vi "2013_04_30 Each Motor.vi"(6 "Temp On":dbl=1.0, 8 "Motor #":i32=1, 9 "data":waveform(dbl)[](array[waveform]), 10 "File Path":path=path "Durability/.lvm", 11 "Motor Typedef":T1 {"Elec Power In (W)" format="%.3g"; "Efficiency" format="%#_3g%%"; "Mech Pwr Out (W)" format="%.3g"; "Torque (mNm)" format="%.3g"; "Elapsed Time (h)" format="%.1f"; "Supply (V)" format="%.2f"; "RPM" scale=0.0..40000.0 scale format="%#_4p"}) -> (0 "Final Out":dynamicdata(graph), 1 "Counter":dbl, 3 "Motor Typedef Out":T1={"Enabled"=FALSE, "Fail"=FALSE, "RPM"=0.0, "Motor"=enum."Maxon EC6 6V", "ESC"=enum."Phoenix", "Supply (V)"=0.0, "Test ID and Serial #"="", "Comments"="", "Elapsed Time (h)"=0.0, "Counter"=0.0, "Torque (mNm)"=0.0, "Mech Pwr Out (W)"=0.0, "Efficiency"=0.0, "Elec Power In (W)"=0.0} {"Elec Power In (W)" format="%.3g"; "Efficiency" format="%#_3g%%"; "Mech Pwr Out (W)" format="%.3g"; "Torque (mNm)" format="%.3g"; "Elapsed Time (h)" format="%.1f"; "Supply (V)" format="%.2f"; "RPM" scale=0.0..40000.0 scale format="%#_4p"})   [LabVIEW 2013]
uses:
  MotorTypeDef.ctl
  <vilib>/express/express shared/transition.llb/Dynamic To Waveform Array.vi
  <vilib>/express/express signal manip/GetorSetDDTAttributes/Set DDT Attributes/SetT0.vi
  <vilib>/express/express shared/transition.llb/Waveform Array To Dynamic.vi
  <vilib>/express/express signal manip/GetorSetDDTAttributes/Set DDT Attributes/Set DDT Properties.xnode
panel:
  in  "error in (no error)":errorcluster
  out "error out":errorcluster
  out "Saving Data":bool
  # "Enable"
  # "Fail"
  # "Enable"
  # "Fail"
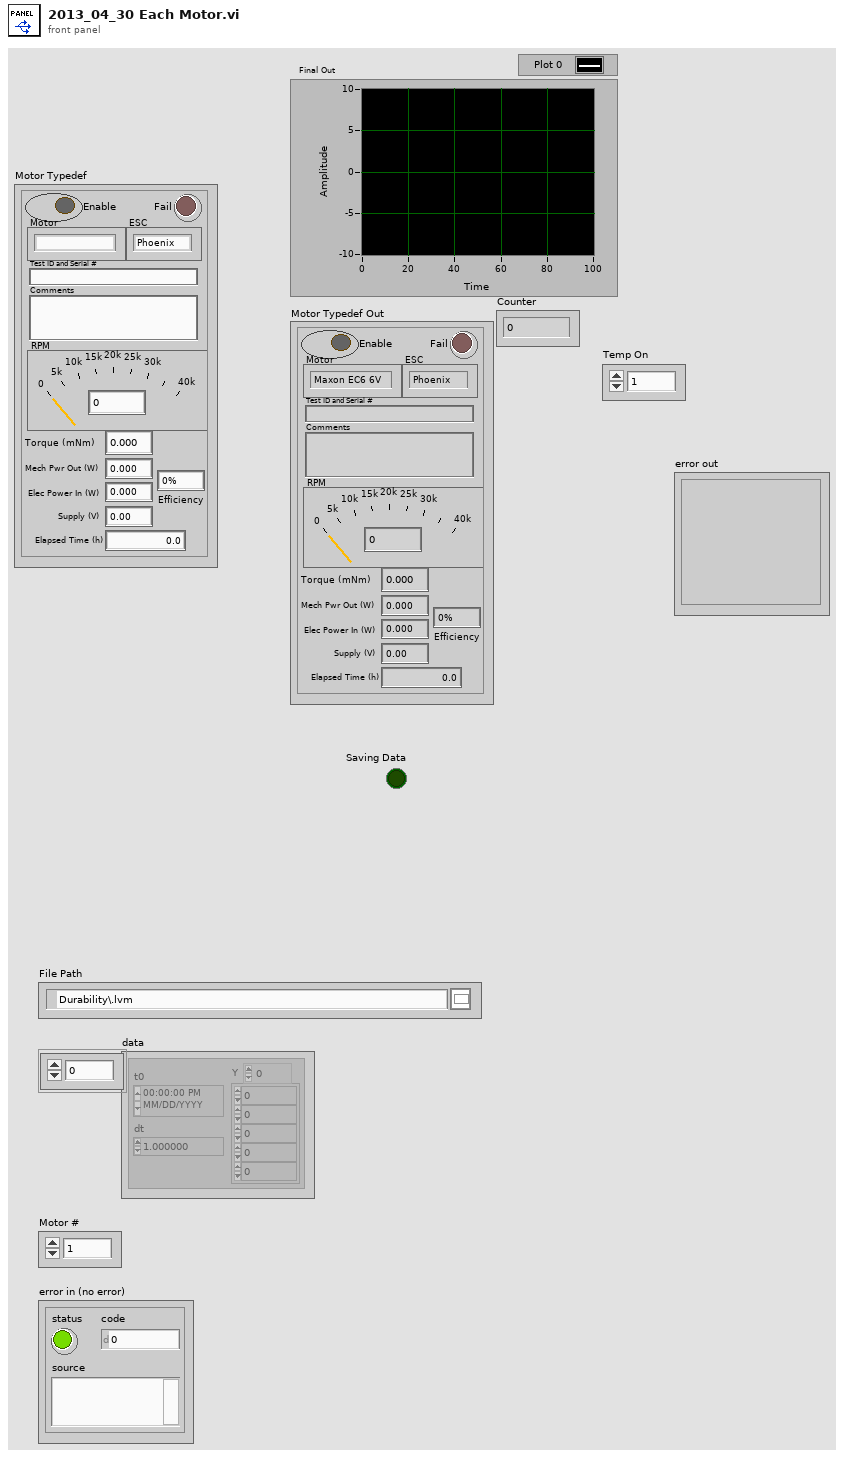
[diagram p1: front panel]
types:
  T1 = typedef "MotorTypeDef.ctl" = cluster{"Enabled":bool, "Fail":bool, "RPM":dbl, "Motor":enum16{"", "Maxon EC6 6V", "Maxon EC4 6V", "FH 0620 6V", "FH 0620 12V"}, "ESC":enum16{"Phoenix", "Maxon", "FH 1801"}, "Supply (V)":dbl, "Test ID and Serial #":string, "Comments":string, "Elapsed Time (h)":dbl, "Counter":dbl, "Torque (mNm)":dbl, "Mech Pwr Out (W)":dbl, "Efficiency":dbl, "Elec Power In (W)":dbl}
  T2 = enum16{"", "Maxon EC6 6V", "Maxon EC4 6V", "FH 0620 6V", "FH 0620 12V"}
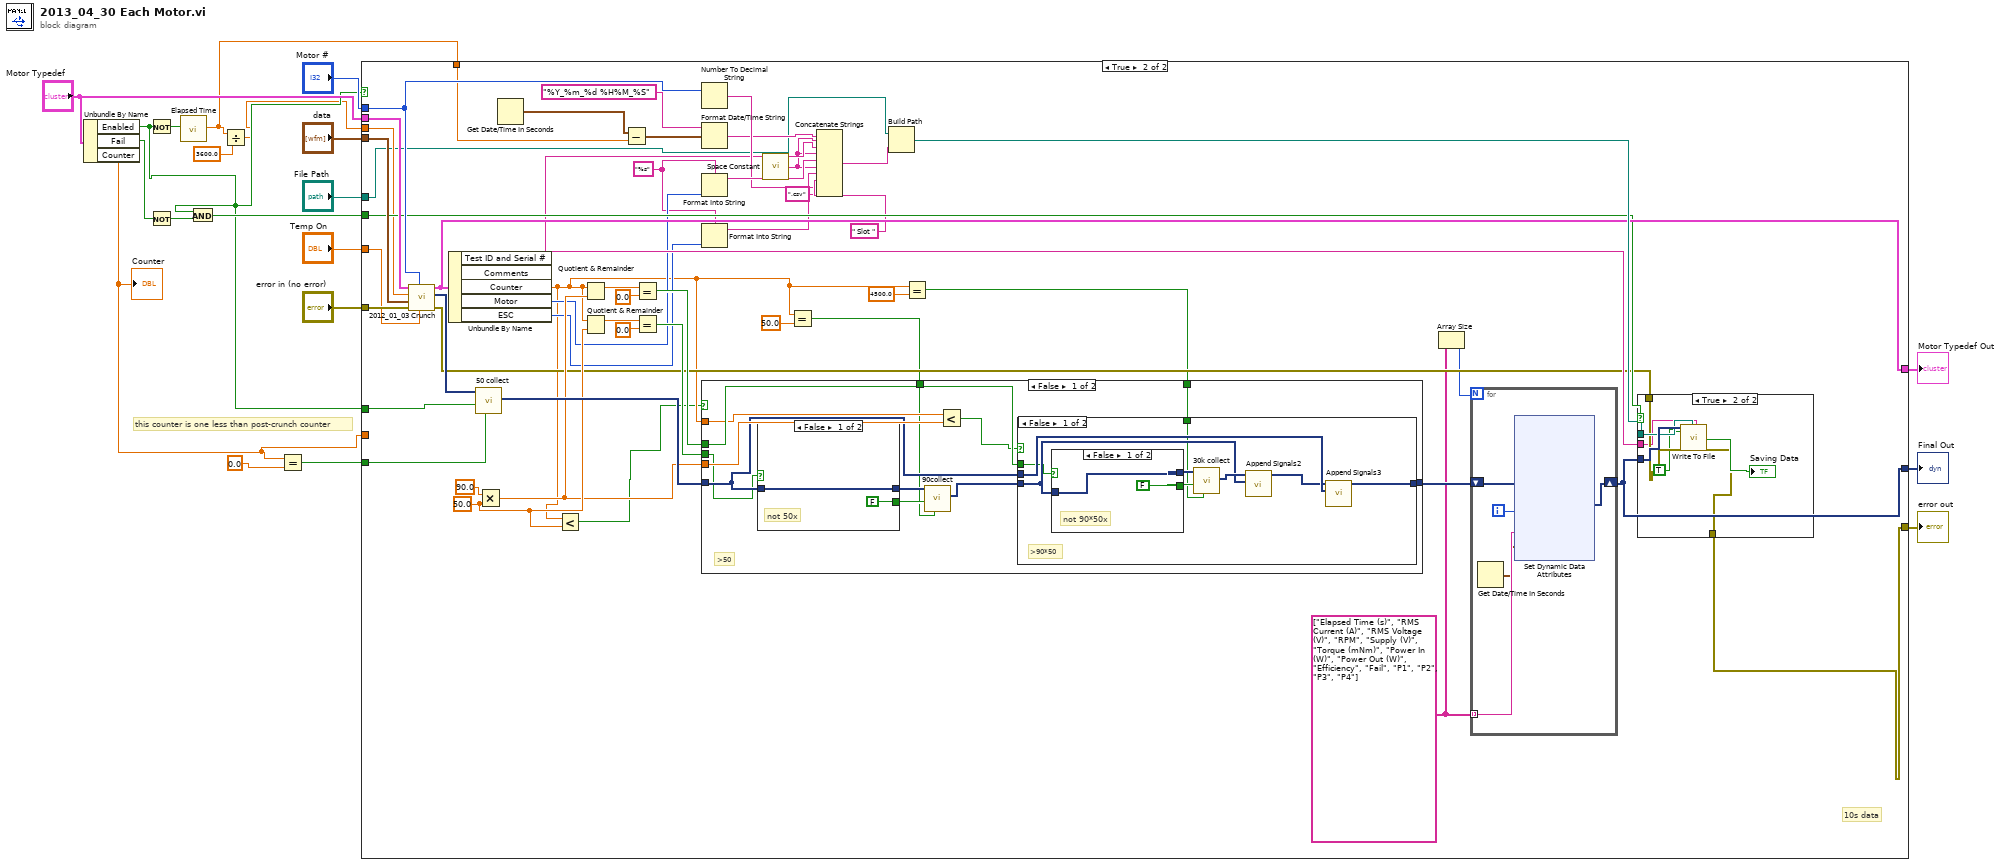
[diagram p0: block diagram]
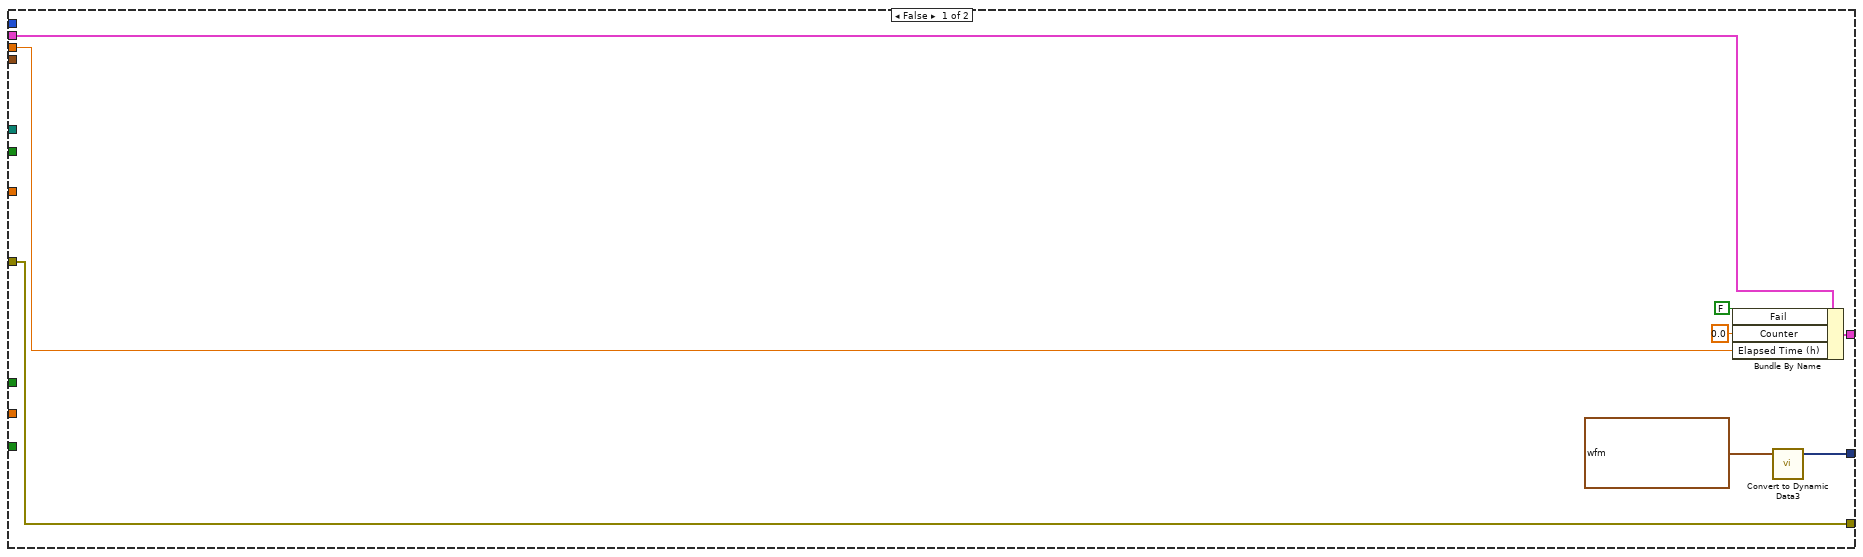
[diagram p2: hidden frame]
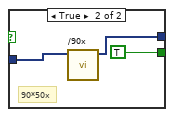
[diagram p3: hidden frame]
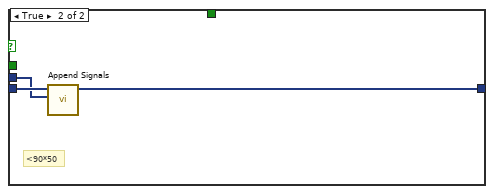
[diagram p4: hidden frame]
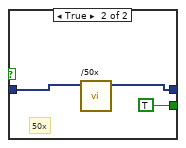
[diagram p5: hidden frame]
diagram:
  # "this counter is one less than post-crunch counter"
  n1 = Unbundle By Name("Motor Typedef") -> ("Enabled"=w4:bool, "Fail"=w11:bool, "Counter"=w5:dbl)
  "Counter" <- w5
  n2 = Not(x=w4) -> (.not. x?=w16:bool)
  n3 = Not(x=w11) -> (.not. x?=w10:bool)
  n4 = call "Elapsed Time"("Reset"=w16) -> ("Elapsed Time (s)"=w1:dbl)  [unwired: 11 in, 7 out]
  n5 = And(x=w4, y=w10) -> (x .and. y?=w9:bool)
  n6 = Divide(x=w1, y=3600.0) -> (x/y=w2:dbl)
  n7 = Equal?(x=w5, y=0.0) -> (x = y?=w7:bool)
  n8 = case shown="True" w4 {
    tunnel: "File Path" -> [_ w33]
    tunnel: [w25 w45] -> w19
    tunnel: "error in (no error)" -> [w25 w80]
    tunnel: "data" -> [_ w79]
    tunnel: [w22 w62] -> w15
    tunnel: w2 -> [w27 w34]
    tunnel: "Motor #" -> [_ w76]
    tunnel: "Motor Typedef" -> [w28 w75]
    tunnel: [w26 w64] -> w12
    tunnel: w9 -> [_ w60]
    tunnel: "Temp On" -> [_ w57]
    tunnel: w7 -> [_ w46]
    tunnel: w5 -> [_ _]
    tunnel: w4 -> [_ w43]
    tunnel: w1 -> [_ w35]
    frame False {
      n9 = Bundle By Name(cluster=w28, "Fail"=FALSE, "Counter"=0.0, "Elapsed Time (h)"=w27) -> (w26:T1)
      n10 = call "Convert to Dynamic Data3"("Waveform"=waveform(dbl) {"t0"=timestamp(0 s since 1904-01-01), "dt"=1.0, "Y"=[]}) -> ("Dynamic Data Type"=w22:dynamicdata)  [unwired: 3 in]
    }
    frame True {
      w53 = "%s" ("format string")
      w29 = string[] ["Elapsed Time (s)", "RMS Current (A)", "RMS Voltage (V)", "RPM", "Supply (V)", "Torque (mNm)", "Power In (W)", "Power Out (W)", "Efficiency", "Fail", "P1", "P2", "P3", "P4"] ("appended array")
      w68 = 50.0 ("y")
      # "10s data"
      n11 = call "2012_01_03 Crunch.vi"("Temp On"=w57, "Motor #"=w76, "error in (no error)"=w80, "data"=w79, "Elapsed Time (h)"=w34, "Motor In"=w75) -> ("error out"=w44:errorcluster, "Dynamic Data Type"=w71:dynamicdata, "Motor Out"=w64:T1)  [unwired: 3 in]
      n12 = Unbundle By Name(w64) -> ("Test ID and Serial #"=w49:string, "Comments"=w77:string, "Counter"=w40:dbl, "Motor"=w56:T2, "ESC"=w52:enum16{"Phoenix", "Maxon", "FH 1801"})
      n13 = call "50 collect"("Reset"=w46, "Enable"=w43, "Signals"=w71) -> ("Collected Signals"=w69:dynamicdata)  [unwired: 7 in, 1 out]
      n14 = Multiply(x=90.0 ("y"), y=w68) -> (x*y=w63:dbl)
      n15 = Get Date/Time In Seconds() -> (seconds since 1Jan1904=w36:timestamp)
      n16 = Less?(x=w40, y=w68) -> (x < y?=w37:bool)
      n17 = Quotient & Remainder(x=w40, y=w63) -> (x-y*floor(x/y)=w67:dbl)  [unwired: 1 out]
      n18 = Quotient & Remainder(x=w40, y=w68) -> (x-y*floor(x/y)=w73:dbl)  [unwired: 1 out]
      n19 = Subtract(x=w36, y=w35) -> (x-y=w59:timestamp)
      n20 = Equal?(x=w67, y=0.0) -> (x = y?=w65:bool)
      n21 = Equal?(x=w73, y=0.0) -> (x = y?=w70:bool)
      n22 = Number To Decimal String(number=w76) -> (decimal integer string=w50:string)  [unwired: 1 in]
      n23 = Format Date/Time String(time format string (%c)="%Y_%m_%d %H%M_%S", seconds (now)=w59) -> (date/time string=w47:string)  [unwired: 1 in]
      n24 = Format Into String(format string=w53, w56) -> (resulting string=w55:string)  [unwired: 2 in, 1 out]
      n25 = Format Into String(format string=w53, w52) -> (resulting string=w54:string)  [unwired: 2 in, 1 out]
      n26 = call <vilib>:"Space Constant.vi"() -> ("String"=w48:string)
      n27 = Equal?(x=w40, y=50.0) -> (x = y?=w41:bool)
      n28 = Concatenate Strings(w47, w48, w49, w48, w55, w48, w54, " Slot " ("string"), w50, ".csv" ("string")) -> (w32:string)
      n29 = Build Path(base path=w33, name or relative path=w32) -> (appended path=w78:path)
      n30 = Equal?(x=w40, y=4500.0) -> (x = y?=w38:bool)
      n31 = case shown="False" w37 {
        tunnel: w70 -> [w104 _]
        tunnel: w69 -> [w110 w137]
        tunnel: [w109 w137] -> w61
        tunnel: w65 -> [w113 _]
        tunnel: w40 -> [w108 _]
        tunnel: w63 -> [w112 _]
        tunnel: w41 -> [w106 _]
        tunnel: w38 -> [w105 _]
        frame False {
          # ">50"
          n32 = case shown="False" w104 {
            tunnel: w110 -> [w133 w136]
            tunnel: [w133 w134] -> w114
            tunnel: [FALSE ("x = y?") TRUE ("x = y?")] -> w107
            frame False {
              # "not 50x"
            }
            frame True {
              # "50x"
              n33 = call "/50x"("Signals"=w136) -> ("Mean"=w134:dynamicdata)  [unwired: 8 in, 2 out]
            }
          }
          n34 = call "90collect"("Reset"=w106, "Enable"=w107, "Signals"=w114) -> ("Collected Signals"=w111:dynamicdata)  [unwired: 7 in, 1 out]
          n35 = Less?(x=w108, y=w112) -> (x < y?=w103:bool)
          n36 = case shown="False" w103 {
            tunnel: w113 -> [w115 _]
            tunnel: w111 -> [w117 w131]
            tunnel: w110 -> [w121 w130]
            tunnel: [w118 w129] -> w109
            tunnel: w105 -> [w116 _]
            frame False {
              # ">90*50"
              n37 = case shown="False" w115 {
                tunnel: w117 -> [w125 w128]
                tunnel: [w125 w127] -> w123
                tunnel: [FALSE ("x = y?") TRUE ("x = y?")] -> w122
                frame False {
                  # "not 90*50x"
                }
                frame True {
                  # "90*50x"
                  n38 = call "/90x"("Signals"=w128) -> ("Mean"=w127:dynamicdata)  [unwired: 8 in, 2 out]
                }
              }
              n39 = call "30k collect"("Reset"=w116, "Enable"=w122, "Signals"=w123) -> ("Collected Signals"=w119:dynamicdata)  [unwired: 7 in, 1 out]
              n40 = call "Append Signals2"("Input Signal B"=w117, "Input Signal A"=w119) -> ("Appended Signals"=w120:dynamicdata)  [unwired: 8 in, 1 out]
              n41 = call "Append Signals3"("Input Signal B"=w121, "Input Signal A"=w120) -> ("Appended Signals"=w118:dynamicdata)  [unwired: 8 in, 1 out]
            }
            frame True {
              # "<90*50"
              n42 = call "Append Signals"("Input Signal B"=w130, "Input Signal A"=w131) -> ("Appended Signals"=w129:dynamicdata)  [unwired: 8 in, 1 out]
            }
          }
        }
        frame True {
          # "<50"
        }
      }
      n43 = Array Size(array=w29) -> (size(s)=w30:i32)
      n44 = for {
        N: w30 -> [_]
        tunnel: w29 -> [w83] mode=indexing
        shift-right: [w84] -> w62
        shift-left: w61 -> [w82]
        i -> [w85]
        n45 = Get Date/Time In Seconds() -> (seconds since 1Jan1904=w81:timestamp)
        n46 = xnode "Set Dynamic Data Attributes"("Signals In"=w82, "Signal Index"=w85, "Signal Name"=w83, "Timestamp"=w81) -> ("Signals Out"=w84:dynamicdata)  [unwired: 1 in, 1 out]
      }
      n47 = case shown="True" w60 {
        tunnel: w62 -> [_ w145]
        tunnel: w78 -> [_ w144]
        tunnel: w77 -> [_ w140]
        tunnel: [w138 w142] -> w45
        tunnel: w44 -> [w138 w141]
        frame False {
        }
        frame True {
          n48 = call "Write To File"("Signals"=w145, "Reset"=TRUE, "error in (no error)"=w141, "Filename"=w144, "Comment"=w140) -> ("Saving Data"=→"Saving Data":bool, "error out"=w142:errorcluster)  [unwired: 12 in, 1 out]
        }
      }
    }
  }
  "error out" <- w19
  "Final Out" <- w15
  "Motor Typedef Out" <- w12
